vi "Questionable Temperature Event Enable Query.vi"(0 "VISA resource name":refnum<visa-resource-name>, 11 "error in (no error)":errorcluster) -> (4 "VISA resource name out":refnum<visa-resource-name>, 6 "Questionable Temperature Event Enable":T1, 15 "error out":errorcluster)   [LabVIEW 2018, in "XP Power PLS600.lvlib"]
doc: "Queries the Questionable Event Enable register. Returns the decimal value of binary-weighted sum of bits.\n\nThe Questionable Temperature Event Enable Register consists of the following 2 bits.\n\nBit 0: Output Board Over-Temp\nBit 1: Primary Board Over-Temp"
uses:
  XP Power PLS600.lvlib
panel:
  # "Bit 0:  Output Board Over-Temp\nBit 1:  Primary Board Over-Temp"
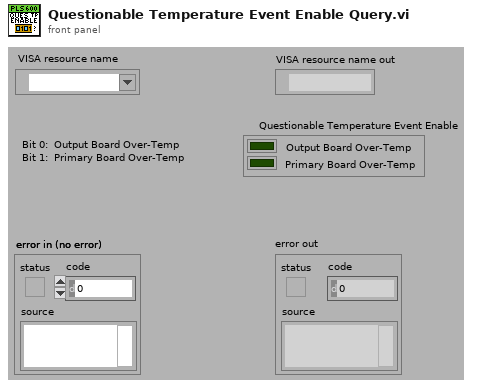
[diagram p1: front panel]
types:
  T1 = cluster{"Output Board Over-Temp":bool, "Primary Board Over-Temp":bool}
  T2 = cluster{"Boolean array[0]":bool, "Boolean array[1]":bool}
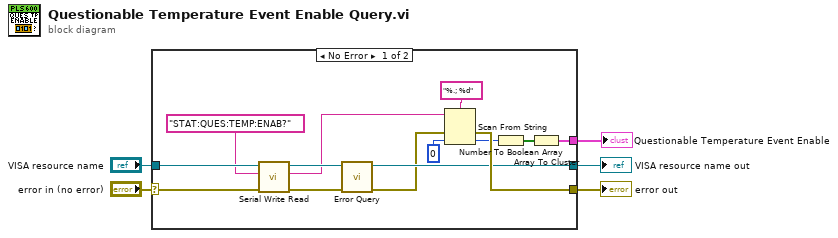
[diagram p0: block diagram]
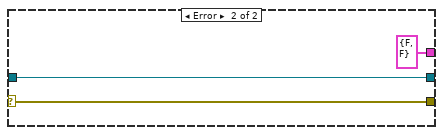
[diagram p2: hidden frame]
diagram:
  n1 = case shown="No Error" "error in (no error)" {
    selector: "error in (no error)" -> [w10 w22]
    tunnel: [w16 T2 {"Boolean array[0]"=FALSE, "Boolean array[1]"=FALSE} ("Boolean array")] -> w1
    tunnel: "VISA resource name" -> [w11 w21]
    tunnel: [w8 w21] -> w4
    tunnel: [w15 w22] -> w3
    frame No Error {
      n2 = call "Serial Write Read.vi"("error in (no error)"=w10, "Write Buffer"="STAT:QUES:TEMP:ENAB?" ("Command to Send (empty)"), "VISA resource name"=w11) -> ("error out"=w13:errorcluster, "Read Buffer"=w6:string, "VISA resource name out"=w12:refnum<visa-resource-name>)  [unwired: 6 in]
      n3 = call "Error Query.vi"("error in (no error)"=w13, "VISA resource name"=w12) -> ("error out"=w7:errorcluster, "VISA resource name out"=w8:refnum<visa-resource-name>)  [unwired: 6 in, 2 out]
      n4 = Scan From String(format string="%.; %d" ("Format String"), input string=w6, error in=w7, default 1=u16 0 ("default value 1")) -> (error out=w15:errorcluster, output 1=w14:u16)  [unwired: 1 in, 2 out]
      n5 = Number To Boolean Array(number=w14) -> (Boolean array=w17:bool[])
      n6 = Array To Cluster(array=w17) -> (cluster=w16:T2)
    }
    frame Error {
    }
  }
  "error out" <- w3
  "VISA resource name out" <- w4
  "Questionable Temperature Event Enable" <- w1
